vi "Display Settings.vi"(11 "ConfigurationThisComponent in":refnum<class "Settings.lvclass">) -> (3 "ConfigurationThisComponent out":refnum<class "Settings.lvclass">)   [LabVIEW 2016, in "Settings.lvclass"]
uses:
  Settings.lvclass
  Typedefs/LogPath.ctl
  Typedefs/ConnectionSettings.ctl
  Typedefs/M1M3SupportEUI_TypeDefs.lvlib
panel:
  in  "ctrlRefArrayUsrEvnt":refnum<user-event>
  in  "ConfigTab":enum32{"Test Data Log", "Connection Settings"}(tab)
  in  "Log Path":T1
  in  "Connection Settings":T2
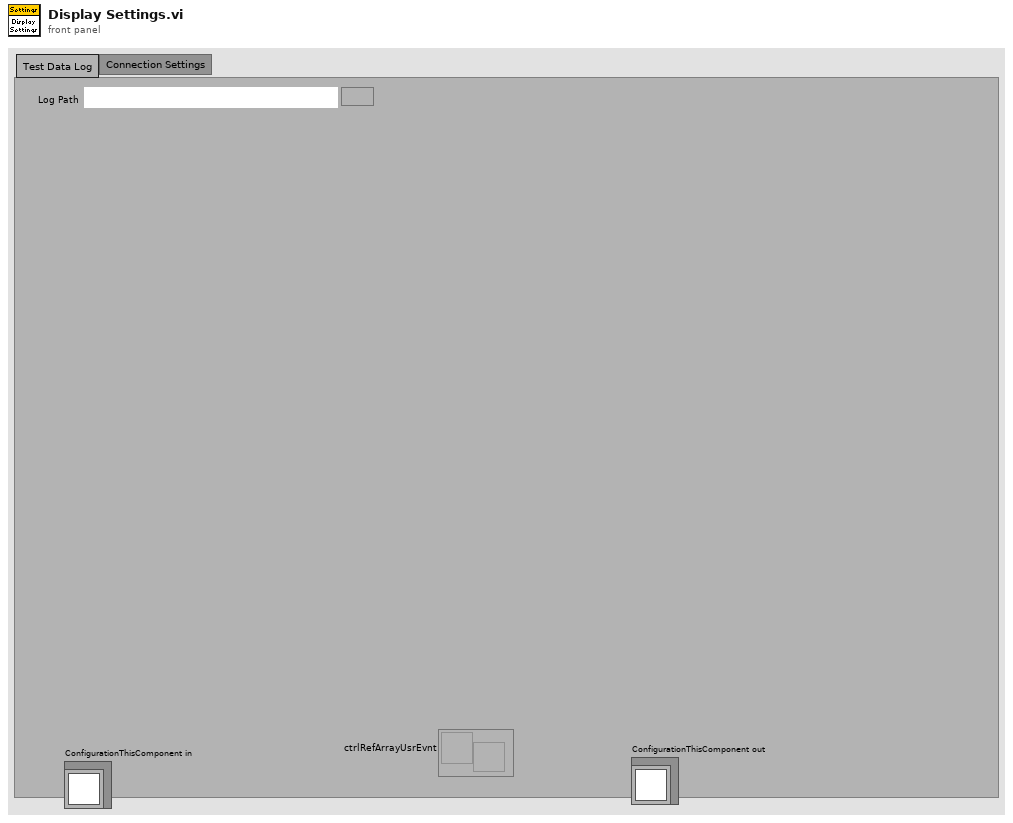
[diagram p1: front panel]
types:
  T1 = typedef "M1M3SupportEUI_TypeDefs.lvlib/LogPath.ctl" = path
  T2 = typedef "M1M3SupportEUI_TypeDefs.lvlib/ConnectionSettings.ctl" = cluster{"ILC Port":refnum<visa-resource-name>}
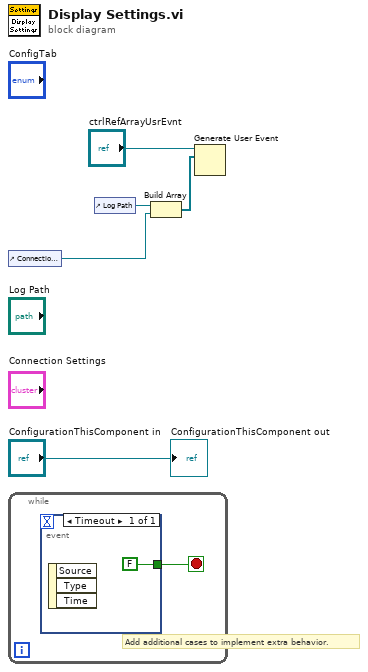
[diagram p0: block diagram]
diagram:
  n1 = control-ref of="Connection Settings"() -> (w1:refnum<vi>)
  n2 = while {
    stop <- w6 stop-if-true
    # "Add additional cases to implement extra behavior."
    n3 = event shown="[0] Timeout" {
      selector: _ -> [_]
      dyn-events: _ -> [_]
      timeout: _ -> [_]
      tunnel: [FALSE] -> w6
      event Timeout {
        n4 = event-data() -> ()  [unwired: 1 in, 3 out]
      }
    }
  }
  n5 = control-ref of="Log Path"() -> (w2:refnum<vi>)
  n6 = Build Array(w2, w1) -> (w3:refnum<vi>[])
  n7 = Generate User Event(user event="ctrlRefArrayUsrEvnt", event data cluster=w3) -> ()  [unwired: 2 in, 2 out]
  "ConfigurationThisComponent out" <- "ConfigurationThisComponent in"
